vi "Stop Audio Device.vi"(8 "error in (no error)":errorcluster, 11 "Audio Device Refnum In":T1) -> (0 "error out":errorcluster, 3 "Audio Device Refnum Out":T1)   [LabVIEW 2020, in "G-Audio.lvlib"]
doc: "Stop the audio device playback or capture.\n\nStopping does not clear any buffered data. Resume device playback / capture with Start Audio Device.vi."
uses:
  G-Audio.lvlib
  Controls/Audio Device Refnum.ctl
  <vilib>/Utility/error.llb/Error Cluster From Error Code.vi
  lib/g_audio_32.dll
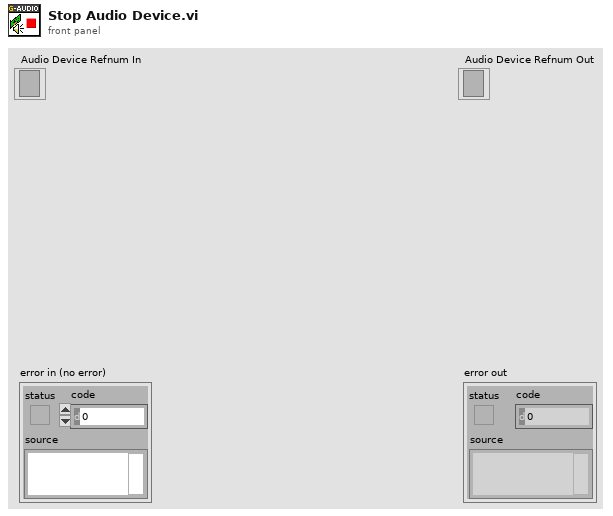
[diagram p1: front panel]
types:
  T1 = typedef "G-Audio.lvlib/Audio Device Refnum.ctl" = refnum<file>
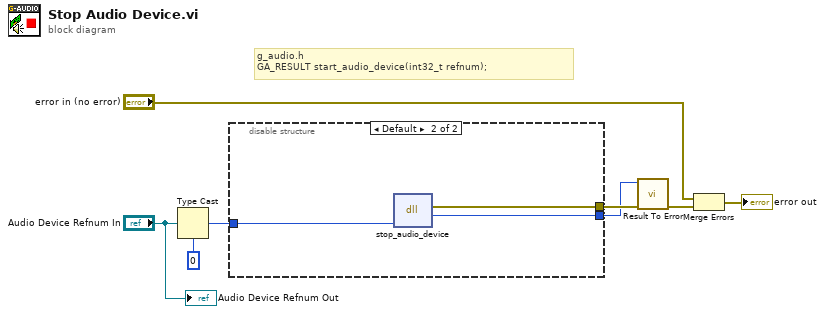
[diagram p0: block diagram]
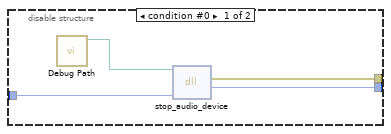
[diagram p2: hidden frame]
diagram:
  # "g_audio.h\nGA_RESULT start_audio_device(int32_t refnum);"
  n1 = Type Cast(type=0, x="Audio Device Refnum In") -> (*(type *) &x=w5:i32)
  n2 = disable-structure shown="Default" {
    disable-tunnel: [w11 w15] -> w8
    disable-tunnel: [w10 w14] -> w7
    disable-tunnel: w5 -> [w9 w13]
    frame condition #0 {
      n3 = call "Debug Path.vi"() -> ("Debug Path"=w12:path)  [unwired: 11 in]
      n4 = dll-call lib="?" fn="stop_audio_device"(path in=w12, "refnum"=w9) -> (error out=w11:errorcluster, "result"=w10:i32)  [unwired: 3 in, 1 out]
    }
    frame condition #1 (active) {
      n5 = dll-call lib="C:/github/dataflowg/g-audio/src/LabVIEW/G-Audio/lib/g_audio_*.*" fn="stop_audio_device"("refnum"=w13) -> (error out=w15:errorcluster, "result"=w14:i32)  [unwired: 4 in, 1 out]
    }
  }
  n6 = call "Result To Error.vi"("error in (no error)"=w8, "Result Code"=w7) -> ("error out"=w2:errorcluster)  [unwired: 9 in]
  n7 = Merge Errors("error in (no error)", w2) -> (→"error out":errorcluster)
  "Audio Device Refnum Out" <- "Audio Device Refnum In"
